vi "Flipper Control.vi"(1 "Flipper VBus in":dbl, 2 "FlipperAtPlace":bool, 3 "InFlipper":bool, 4 "FrisbiInCannon":bool) -> (0 "Flipper VBus out":dbl)   [LabVIEW 2012]
panel:
  # "Cannon"
  # "InFlipper"
  # "FlipperAtPlace"
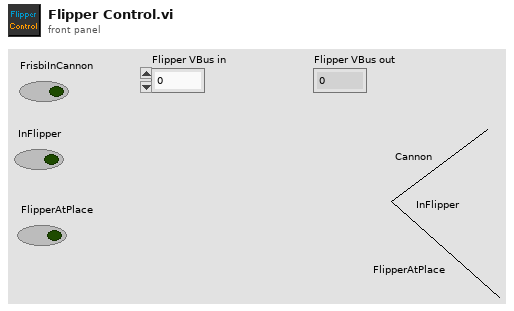
[diagram p1: front panel]
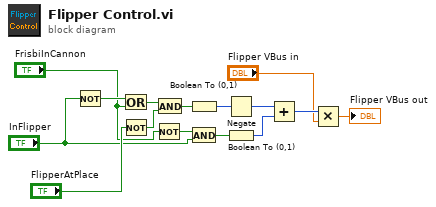
[diagram p0: block diagram]
diagram:
  n1 = Not(x="InFlipper") -> (.not. x?=w12:bool)
  n2 = Or(x=w12, y="FrisbiInCannon") -> (x .or. y?=w13:bool)
  n3 = Not(x="FlipperAtPlace") -> (.not. x?=w14:bool)
  n4 = Not(x="FrisbiInCannon") -> (.not. x?=w8:bool)
  n5 = And(x=w13, y=w14) -> (x .and. y?=w11:bool)
  n6 = Boolean To (0,1)(Boolean=w11) -> (0, 1=w10:i16)
  n7 = And(x=w8, y="InFlipper") -> (x .and. y?=w6:bool)
  n8 = Negate(x=w10) -> (-x=w5:i16)
  n9 = Boolean To (0,1)(Boolean=w6) -> (0, 1=w4:i16)
  n10 = Add(x=w5, y=w4) -> (x+y=w3:i16)
  n11 = Multiply(x=w3, y="Flipper VBus in") -> (x*y=→"Flipper VBus out":dbl)
